vi "Write Z_state.vi"(8 "error in (no error)":errorcluster, 10 "Heating.lvlib:HE_Z_state.lvclass":refnum<class "HE_Z_state.lvclass">, 11 "HE_state in":refnum<class "HE_state_v2.lvclass">) -> (0 "error out":errorcluster, 3 "HE_state out":refnum<class "HE_state_v2.lvclass">)   [LabVIEW 2019]
uses:
  HE_state_v2.lvclass
  C:/my_projects/projects/Algorithms/Labview/19/Heating/heating1/Z_state_v2/HE_Z_state_v2.lvclass
  C:/my_projects/projects/Algorithms/Labview/19/Heating/heating1/ZM_state/HE_ZM_state.lvclass
  C:/my_projects/projects/Algorithms/Labview/19/Sequence/State/State.lvclass
  Z_state/HE_Z_state.lvclass
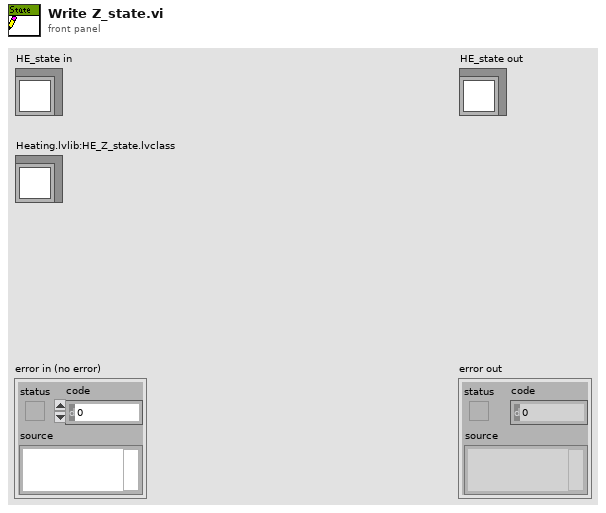
[diagram p1: front panel]
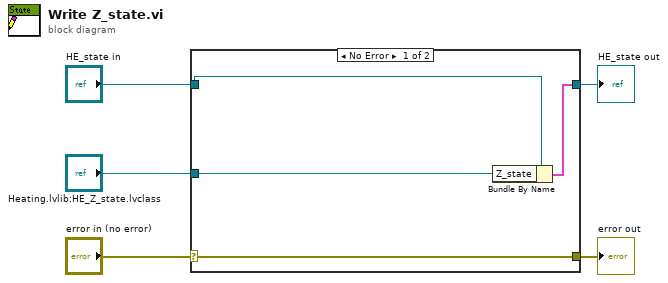
[diagram p0: block diagram]
diagram:
  n1 = case shown="No Error" "error in (no error)" {
    selector: "error in (no error)" -> [w9 w10]
    tunnel: [w9 w10] -> w4
    tunnel: [w7 w11] -> w2
    tunnel: "HE_state in" -> [w8 w11]
    tunnel: "Heating.lvlib:HE_Z_state.lvclass" -> [w6 _]
    frame No Error {
      n2 = Bundle By Name(cluster=w8, "Z_state"=w6) -> (w7:cluster{})
    }
    frame Error {
    }
  }
  "error out" <- w4
  "HE_state out" <- w2
